vi "GetParam.vi"(8 "error in (no error)":errorcluster caption="entrée d'erreur (pas d'erreur)", 11 "Moons.lvclass":refnum<class "Moons.lvclass">) -> (0 "error out":errorcluster caption="sortie d'erreur", 2 "make_moons":T1={"n_samples"="100", "shuffle"=TRUE, "noise"=-1.0, "random_state"=-1, "Returns"="X"} {"noise" min=-1.0; "random_state" min=-1}, 3 "Moons.lvclass":refnum<class "Moons.lvclass">)   [LabVIEW 2020, in "Moons.lvclass"]
doc: "Get Parameters"
uses:
  Moons.lvclass
  Moons.lvclass/Moons.ctl
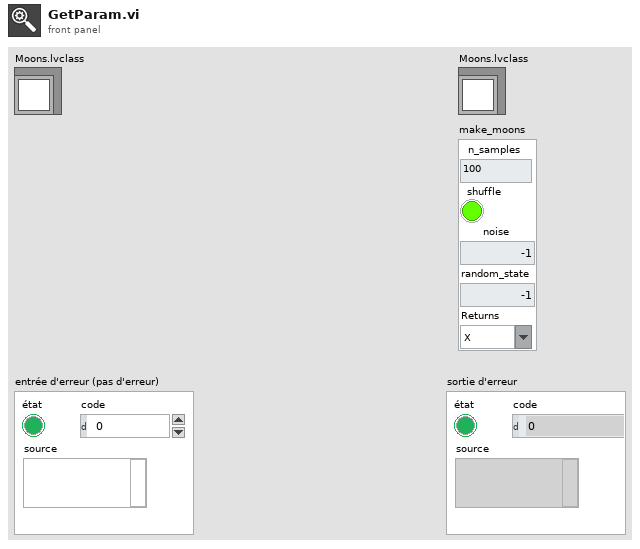
[diagram p1: front panel]
types:
  T1 = cluster{"n_samples":string, "shuffle":bool, "noise":dbl, "random_state":i32, "Returns":string}
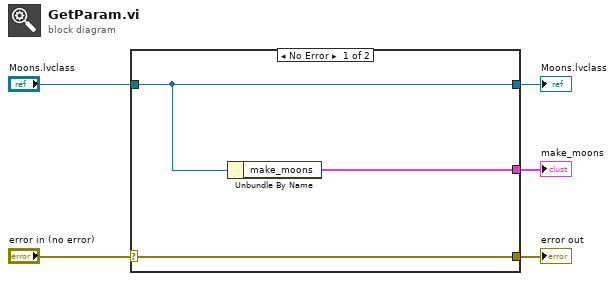
[diagram p0: block diagram]
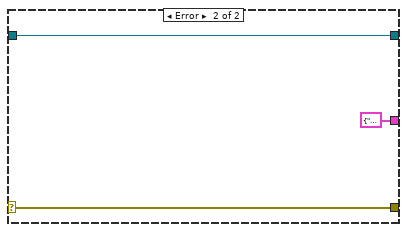
[diagram p2: hidden frame]
diagram:
  n1 = case shown="No Error" "error in (no error)" {
    selector: "error in (no error)" -> [w8 w10]
    tunnel: [w8 w10] -> w4
    tunnel: [w7 w11] -> w2
    tunnel: "Moons.lvclass" -> [w7 w11]
    tunnel: [w6 T1 {"n_samples"="", "shuffle"=FALSE, "noise"=0.0, "random_state"=0, "Returns"=""} ("make_moons")] -> w1
    frame No Error {
      n2 = Unbundle By Name(w7) -> ("make_moons"=w6:T1)
    }
    frame Error {
    }
  }
  "error out" <- w4
  "Moons.lvclass" <- w2
  "make_moons" <- w1
